vi "stop allconnections and close refs.vi"(11 "Comms data":T1) -> ()   [LabVIEW 2018]
uses:
  comms data.ctl
  Type Defs/generic incident.ctl
  Github/ICL-LabVIEW_General/Scanivalve API project/full interface/polymorphic/scanivalveConfig.ctl
  Github/ICL-LabVIEW_General/Scanivalve API project/full interface/listS.ctl
  Github/ICL-LabVIEW_General/Scanivalve API project/full interface/listC.ctl
  Github/ICL-LabVIEW_General/Scanivalve API project/full interface/listSG.ctl
  Github/ICL-LabVIEW_General/Scanivalve API project/full interface/chan1.ctl
  <vilib>/dex/Flush And Wait Empty Condition.ctl
  Github/ICL-LabVIEW_General/Main Controller SVE/Controller Data/Cabinet data FGV states.ctl
  Github/ICL-LabVIEW_General/Scanivalve API project/polymorphic vis/close connection with scanivalve.vi
  Github/ICL-LabVIEW_General/Scanivalve API project/Scanivalve API.lvlib
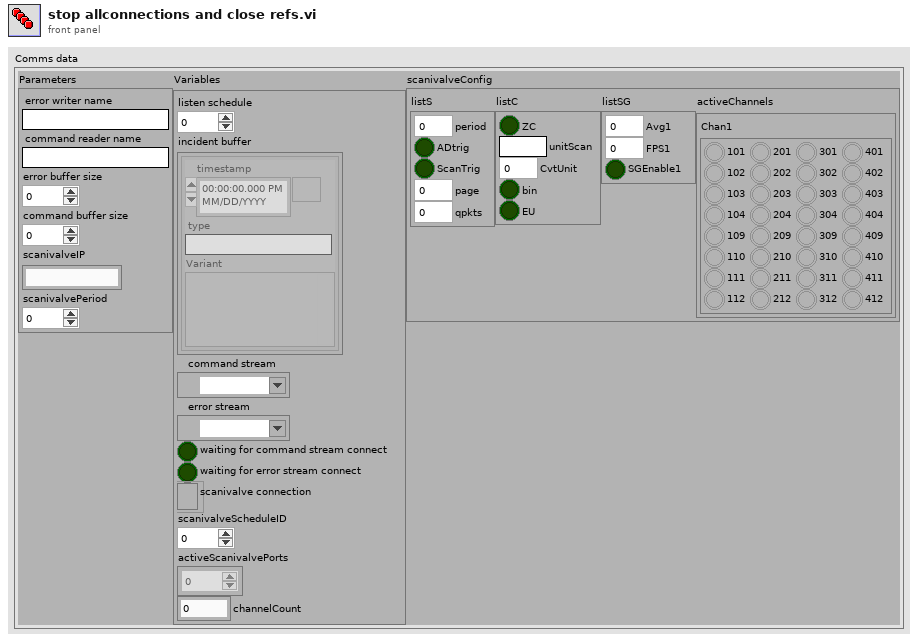
[diagram p1: front panel]
types:
  T1 = typedef "comms data.ctl" = cluster{"Parameters":cluster{"error writer name":string, "command reader name":string, "error buffer size":i32, "command buffer size":i32, "scanivalveIP":string, "scanivalvePeriod":u16}, "Variables":cluster{"listen schedule":u32, "incident buffer":T2[], "command stream":refnum<k21>, "error stream":refnum<k21>, "waiting for command stream connect":bool, "waiting for error stream connect":bool, "scanivalve connection":refnum<k5>, "scanivalveScheduleID":u32, "activeScanivalvePorts":i32[], "channelCount":i16}, "scanivalveConfig":T3}
  T2 = typedef "generic incident.ctl" = cluster{"timestamp":timestamp, "type":string, "Variant":variant}
  T3 = typedef "scanivalveConfig.ctl" = cluster{"listS":T4, "listC":T5, "listSG":T6, "activeChannels":T7}
  T4 = typedef "listS.ctl" = cluster{"period":u16, "ADtrig":bool, "ScanTrig":bool, "page":u16, "qpkts":u16}
  T5 = typedef "listC.ctl" = cluster{"ZC":bool, "unitScan":string, "CvtUnit":dbl, "bin":bool, "EU":bool}
  T6 = typedef "listSG.ctl" = cluster{"Avg1":u16, "FPS1":u16, "SGEnable1":bool}
  T7 = typedef "chan1.ctl" = cluster{"Chan1":cluster{"101":bool, "102":bool, "103":bool, "104":bool, "109":bool, "110":bool, "111":bool, "112":bool, "201":bool, "202":bool, "203":bool, "204":bool, "209":bool, "210":bool, "211":bool, "212":bool, "301":bool, "302":bool, "303":bool, "304":bool, "309":bool, "310":bool, "311":bool, "312":bool, "401":bool, "402":bool, "403":bool, "404":bool, "409":bool, "410":bool, "411":bool, "412":bool}}
  T8 = typedef "Cabinet data FGV states.ctl" = enum16{"connect", "read", "disconnect"}
  T9 = typedef "Flush And Wait Empty Condition.ctl" = u8
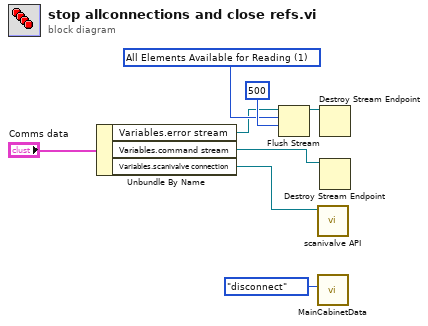
[diagram p0: block diagram]
diagram:
  w7 = T9 1 items=["All Elements Read From Stream", "All Elements Available for Reading"] ("wait condition")
  n1 = Unbundle By Name("Comms data") -> ("Variables.error stream"=w5:refnum<k21>, "Variables.command stream"=w3:refnum<k21>, "Variables.scanivalve connection"=w1:refnum<k5>)
  n2 = Flush Stream(9:500 ("timeout in ms (-1)"), 10:w7, 11:w5) -> (3:w6:refnum<k21>)  [unwired: 1 in, 2 out]
  n3 = call-poly "scanivalve API.vi"("scanivalve connection in"=w1) -> ()  [unwired: 10 in, 1 out]
  n4 = call "MainCabinetData.vi"("Action"=Cabinet_data_FGV_states."disconnect") -> ()  [unwired: 8 in, 3 out]
  n5 = Destroy Stream Endpoint(11:w6) -> ()  [unwired: 1 in, 1 out]
  n6 = Destroy Stream Endpoint(11:w3) -> ()  [unwired: 1 in, 1 out]
